vi "PLC test.vi"() -> ()   [LabVIEW 2017]
uses:
  <vilib>/DATA AHEAD/SP7/typedefs/PLC Type.ctl
  <vilib>/DATA AHEAD/SP7/functions/read/read Dint array.vi
  <vilib>/DATA AHEAD/SP7/functions/read/read real array.vi
  <vilib>/DATA AHEAD/SP7/functions/read/read String.vi
  Global/Global 1.vi
  <vilib>/DATA AHEAD/SP7/SP7.lvlib
  <vilib>/DATA AHEAD/SP7/functions/read/read int array.vi
  Global/DATA LOG.vi
  <vilib>/DATA AHEAD/SP7/functions/write/write Dint array.vi
panel:
  out "STRING result Array 2":string[](array[string])
  out "error out":errorcluster
  out "STRING result Array":string[](array[string])
  out "DINT result array":i32[](array[numeric])
  out "REAL result array":sgl[](array[numeric])
  out "IP address":string="192.168.0.10"
  out "error out 2":errorcluster
  in  "stop":bool
  out "PLC 1":bool
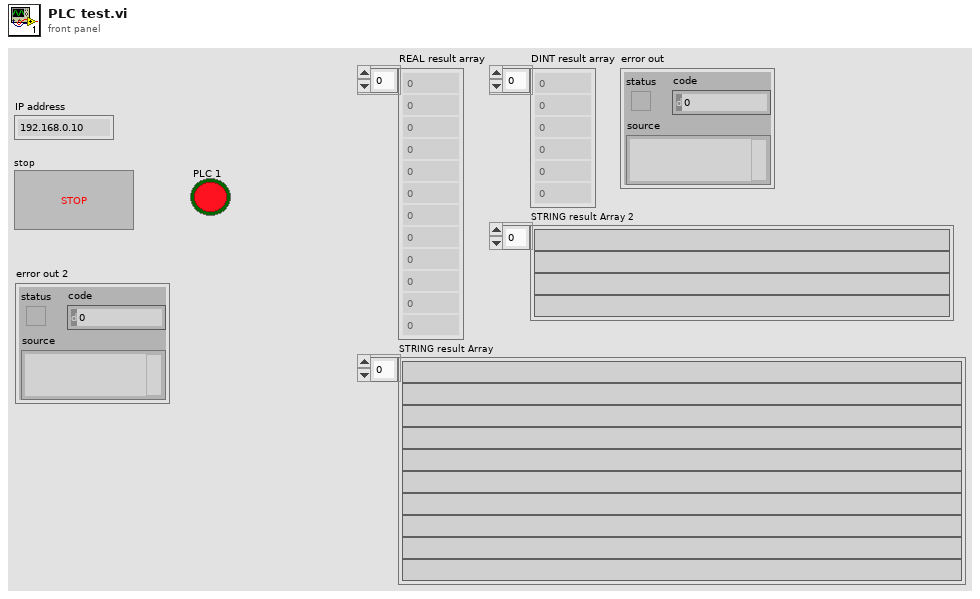
[diagram p1: front panel]
types:
  T1 = typedef "SP7.lvlib/PLC Type.ctl" = enum16{"S7 200", "S7 300/400", "S7 1200", "S7 1500", "LOGO!8"}
  T2 = typedef "SP7.lvlib/S7 Connection.ctl" = cluster{"TCP Connection Ref":refnum<k5>, "IP address":string, "timeout ms":i32, "Connected?":bool, "PLC Type":T1, "Rack S7 400":u8, "Slot S7 400":u8, "PDU Size":u16, "connection semaphore":T3}
  T3 = typedef "Semaphore RefNum" = refnum<k1>
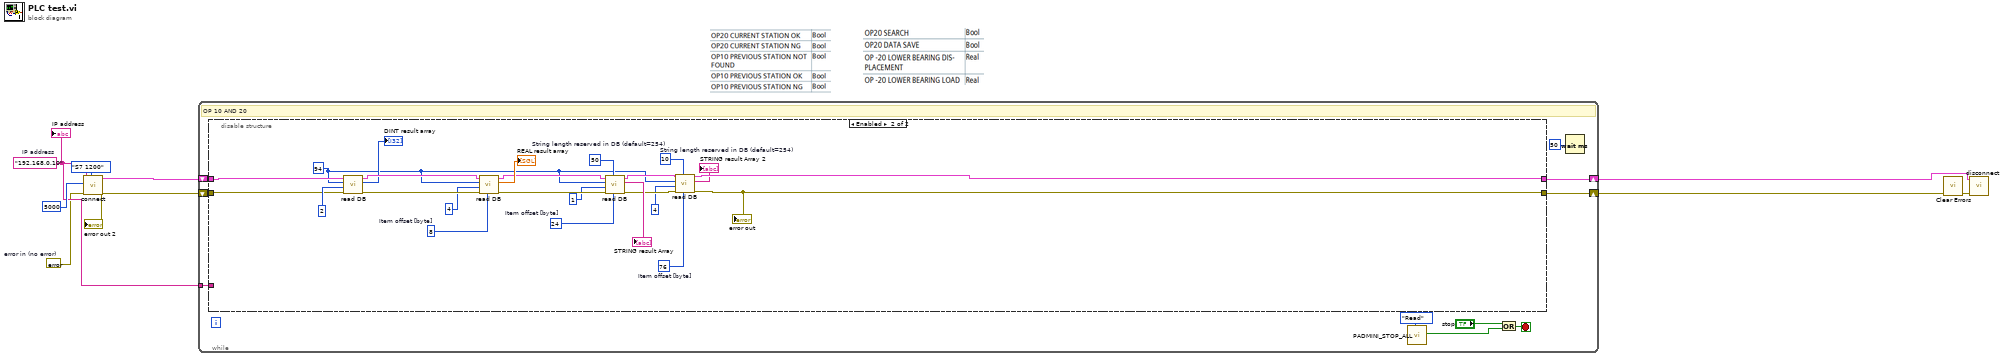
[diagram p0: block diagram]
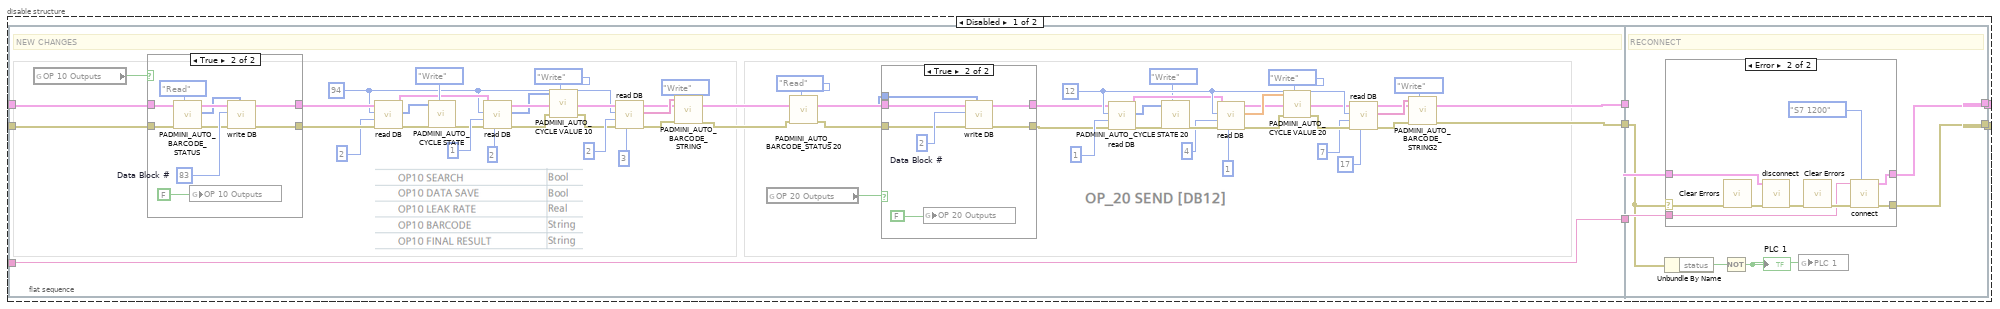
[diagram p2: hidden frame]
diagram:
  w1 = errorcluster {"status"=FALSE, "code"=0, "source"=""}  # error in (no error)
  w2 = "192.168.0.10"  # IP address
  n1 = call <vilib>:"connect.vi"("PLC Type"=PLC_Type."S7 1200" ("PLC Type 2"), "error in (no error)"=w1, "timeout [ms]"=5000, "IP address"=w2) -> ("error out"=w6:errorcluster, "S7 Connection out"=w5:T2)  [unwired: 6 in]
  "error out 2" <- w6
  n2 = while {
    shift-right: [w11] -> w3
    shift-left: w5 -> [w19]
    shift-right: [w17] -> w9
    shift-left: w6 -> [w18]
    tunnel: w2 -> [w10]
    stop <- w12 stop-if-true
    # "OP 10 AND 20"
    n3 = disable-structure shown="Enabled" {
      disable-tunnel: w19 -> [w24 w142]
      disable-tunnel: w18 -> [w23 w141]
      disable-tunnel: [w22 w126] -> w17
      disable-tunnel: [w21 w127] -> w11
      disable-tunnel: w10 -> [w20 _]
      frame Disabled {
        n4 = flat-sequence {
          tunnel: [w30] -> w27
          tunnel: [w29] -> w26
          tunnel: w23 -> [w63]
          tunnel: w24 -> [w80]
          tunnel: [w28] -> w25
          tunnel: w20 -> [w28]
          tunnel: [w105] -> w22
          tunnel: [w104] -> w21
          tunnel: w27 -> [w106]
          tunnel: w26 -> [w102]
          tunnel: w25 -> [w103]
          frame #0 {
            w45 = u16 12 ("Data Block #")
            w70 = u16 94 ("Data Block #")
            # "NEW CHANGES"
            n5 = global read "DATA LOG.vi" "OP 10 Outputs"() -> (w62:bool)
            n6 = case shown="True" w62 {
              tunnel: w80 -> [w91 w100]
              tunnel: [w92 w99] -> w79
              tunnel: [w91 w98] -> w77
              tunnel: w63 -> [w92 w95]
              frame False {
              }
              frame True {
                w101 = u16 83  # Data Block #
                n7 = call "PADMINI_AUTO_BARCODE_STATUS.vi"("Enum"=enum16{"Read", "Write"}."Read", "error in (no error)"=w95) -> ("error out"=w94:errorcluster, "O/P"=w96:i32[])  [unwired: 8 in]
                n8 = global write "DATA LOG.vi" "OP 10 Outputs"(FALSE) -> ()
                n9 = call-poly <vilib>:"write DB.vi"("DINT input array"=w96, "error in (no error)"=w94, "Data Block #"=w101, "S7 Connection in"=w100) -> ("error out"=w99:errorcluster, "S7 Connection out"=w98:T2)  [unwired: 4 in, 2 out]
              }
            }
            n10 = call-poly <vilib>:"read DB.vi"("error in (no error)"=w79, "items #"=u16 2 ("Items # [byte]"), "Data Block #"=w70, "S7 Connection in"=w77) -> ("error out"=w78:errorcluster, "DINT result array"=w75:i32[], "S7 Connection out"=w72:T2)  [unwired: 5 in]
            n11 = call "PADMINI_AUTO_CYCLE STATE.vi"("Enum"=enum16{"Read", "Write"}."Write", "error in (no error)"=w78, "Input"=w75) -> ("error out"=w73:errorcluster)  [unwired: 7 in, 1 out]
            n12 = call-poly <vilib>:"read DB.vi"("Item offset [byte]"=u32 2, "error in (no error)"=w73, "items #"=u16 1 ("Items # [byte]"), "Data Block #"=w70, "S7 Connection in"=w72) -> ("error out"=w60:errorcluster, "Int result array"=w58:i16[], "S7 Connection out"=w71:T2)  [unwired: 4 in]
            n13 = call "PADMINI_AUTO_CYCLE VALUE 10.vi"("Enum"=enum16{"Read", "Write"}."Write", "error in (no error)"=w60, "Input"=w58) -> ("error out"=w59:errorcluster)  [unwired: 7 in, 1 out]
            n14 = call-poly <vilib>:"read DB.vi"("Item offset [byte]"=u32 3, "error in (no error)"=w59, "items #"=u16 2 ("Items # [byte]"), "Data Block #"=w70, "S7 Connection in"=w71) -> ("error out"=w66:errorcluster, "STRING result Array"=w67:string[], "S7 Connection out"=w57:T2)  [unwired: 3 in, 1 out]
            n15 = call "PADMINI_AUTO_BARCODE_STRING.vi"("Enum"=enum16{"Read", "Write"}."Write", "error in (no error)"=w66, "Input"=w67) -> ("error out"=w33:errorcluster)  [unwired: 7 in, 1 out]
            n16 = global read "DATA LOG.vi" "OP 20 Outputs"() -> (w56:bool)
            n17 = call "PADMINI_AUTO_BARCODE_STATUS 20.vi"("Enum"=enum16{"Read", "Write"}."Read", "error in (no error)"=w33) -> ("error out"=w32:errorcluster, "O/P"=w31:i32[])  [unwired: 8 in]
            n18 = case shown="True" w56 {
              tunnel: w57 -> [w82 w86]
              tunnel: [w83 w89] -> w36
              tunnel: [w82 w88] -> w35
              tunnel: w32 -> [w83 w85]
              tunnel: w31 -> [_ w84]
              frame False {
              }
              frame True {
                w90 = u16 2  # Data Block #
                n19 = global write "DATA LOG.vi" "OP 20 Outputs"(FALSE) -> ()
                n20 = call-poly <vilib>:"write DB.vi"("DINT input array"=w84, "error in (no error)"=w85, "Data Block #"=w90, "S7 Connection in"=w86) -> ("error out"=w89:errorcluster, "S7 Connection out"=w88:T2)  [unwired: 4 in, 2 out]
              }
            }
            n21 = call-poly <vilib>:"read DB.vi"("error in (no error)"=w36, "items #"=u16 1 ("Items # [byte]"), "Data Block #"=w45, "S7 Connection in"=w35) -> ("error out"=w38:errorcluster, "DINT result array"=w40:i32[], "S7 Connection out"=w43:T2)  [unwired: 5 in]
            n22 = call "PADMINI_AUTO_CYCLE STATE 20.vi"("Enum"=enum16{"Read", "Write"}."Write", "error in (no error)"=w38, "Input"=w40) -> ("error out"=w42:errorcluster)  [unwired: 7 in, 1 out]
            n23 = call-poly <vilib>:"read DB.vi"("Item offset [byte]"=u32 1, "error in (no error)"=w42, "items #"=u16 4 ("Items # [byte]"), "Data Block #"=w45, "S7 Connection in"=w43) -> ("error out"=w53:errorcluster, "REAL result array"=w55:sgl[], "S7 Connection out"=w44:T2)  [unwired: 4 in]
            n24 = call "PADMINI_AUTO_CYCLE VALUE 20.vi"("Enum"=enum16{"Read", "Write"}."Write", "error in (no error)"=w53, "Input"=w55) -> ("error out"=w54:errorcluster)  [unwired: 7 in, 1 out]
            n25 = call-poly <vilib>:"read DB.vi"("Item offset [byte]"=u32 17, "error in (no error)"=w54, "items #"=u16 7 ("Items # [byte]"), "Data Block #"=w45, "S7 Connection in"=w44) -> ("error out"=w49:errorcluster, "STRING result Array"=w48:string[], "S7 Connection out"=w30:T2)  [unwired: 3 in, 1 out]
            n26 = call "PADMINI_AUTO_BARCODE_STRING2.vi"("Enum"=enum16{"Read", "Write"}."Write", "error in (no error)"=w49, "Input"=w48) -> ("error out"=w29:errorcluster)  [unwired: 7 in, 1 out]
          }
          frame #1 {
            # "RECONNECT"
            n27 = Unbundle By Name(w102) -> ("status"=w108:bool)
            n28 = case shown="Error" w102 {
              selector: w102 -> [w110 w118]
              tunnel: [w109 w115] -> w104
              tunnel: [w110 w116] -> w105
              tunnel: w106 -> [w109 w112]
              tunnel: w103 -> [_ w111]
              frame No Error {
              }
              frame Error {
                n29 = call <vilib>:"Clear Errors.vi"("error in (no error)"=w118) -> ("error out"=w119:errorcluster)  [unwired: 5 in, 1 out]
                n30 = call <vilib>:"disconnect.vi"("error in (no error)"=w119, "S7 Connection in"=w112) -> ("error out"=w117:errorcluster)  [unwired: 8 in, 1 out]
                n31 = call <vilib>:"Clear Errors.vi"("error in (no error)"=w117) -> ("error out"=w114:errorcluster)  [unwired: 5 in, 1 out]
                n32 = call <vilib>:"connect.vi"("PLC Type"=PLC_Type."S7 1200" ("PLC Type 2"), "error in (no error)"=w114, "IP address"=w111) -> ("error out"=w116:errorcluster, "S7 Connection out"=w115:T2)  [unwired: 7 in]
              }
            }
            n33 = Not(x=w108) -> (.not. x?=w107:bool)
            "PLC 1" <- w107
            n34 = global write "Global 1.vi" "PLC 1"(w107) -> ()
          }
        }
      }
      frame Enabled {
        w121 = u32 76  # Item offset [byte]
        w124 = u16 10  # String length reserved in DB (default=254)
        w129 = u16 50  # String length reserved in DB (default=254)
        w131 = u32 24  # Item offset [byte]
        w136 = u32 8  # Item offset [byte]
        w123 = u16 94 ("Data Block #")
        n35 = call-poly <vilib>:"read DB.vi"("error in (no error)"=w141, "items #"=u16 2 ("Items # [byte]"), "Data Block #"=w123, "S7 Connection in"=w142) -> ("error out"=w139:errorcluster, "DINT result array"=→"DINT result array":i32[], "S7 Connection out"=w140:T2)  [unwired: 5 in]
        n36 = call-poly <vilib>:"read DB.vi"("Item offset [byte]"=w136, "error in (no error)"=w139, "items #"=u16 4 ("Items # [byte]"), "Data Block #"=w123, "S7 Connection in"=w140) -> ("error out"=w133:errorcluster, "REAL result array"=→"REAL result array":sgl[], "S7 Connection out"=w134:T2)  [unwired: 4 in]
        n37 = call-poly <vilib>:"read DB.vi"("Item offset [byte]"=w131, "String length reserved in DB (default=254)"=w129, "error in (no error)"=w133, "items #"=u16 1 ("Items # [byte]"), "Data Block #"=w123, "S7 Connection in"=w134) -> ("error out"=w125:errorcluster, "STRING result Array"=→"STRING result Array":string[], "S7 Connection out"=w128:T2)  [unwired: 2 in, 1 out]
        n38 = call-poly <vilib>:"read DB.vi"("Item offset [byte]"=w121, "String length reserved in DB (default=254)"=w124, "error in (no error)"=w125, "items #"=u16 4 ("Items # [byte]"), "Data Block #"=w123, "S7 Connection in"=w128) -> ("error out"=w126:errorcluster, "STRING result Array"=→"STRING result Array 2":string[], "S7 Connection out"=w127:T2)  [unwired: 2 in, 1 out]
        "error out" <- w126
      }
    }
    n39 = call "PADMINI_STOP_ALL.vi"("Enum"=enum16{"Read", "Write"}."Read") -> ("Boolean 2"=w14:bool)  [unwired: 9 in, 1 out]
    n40 = Or(x="stop", y=w14) -> (x .or. y?=w12:bool)
    n41 = Wait (ms)(milliseconds to wait=u32 50) -> ()  [unwired: 1 out]
  }
  n42 = call <vilib>:"Clear Errors.vi"("error in (no error)"=w9) -> ("error out"=w4:errorcluster)  [unwired: 5 in, 1 out]
  n43 = call <vilib>:"disconnect.vi"("error in (no error)"=w4, "S7 Connection in"=w3) -> ()  [unwired: 8 in, 2 out]
  "IP address" <- w2
